vi "DSF.Shared.Configuration.Framework.New Transfer.vi"(8 "error in (no error)":errorcluster, 11 "Framework Configuration in":refnum<class "DSF.Shared.Configuration.Framework.lvclass">) -> (0 "error out":errorcluster, 2 "Transfer Configuration":refnum<class "DSF.Shared.Configuration.Transfer.lvclass">, 3 "Framework Configuration out":refnum<class "DSF.Shared.Configuration.Framework.lvclass">)   [LabVIEW 2016, in "DSF.Shared.lvlib" / "DSF.Shared.Configuration.Framework.lvclass"]
uses:
  DSF.Shared.Configuration.Framework.lvclass
  Transfer/DSF.Shared.Configuration.Transfer.lvclass
  DSF.Shared.Configuration.Framework.lvclass/DSF.Shared.Configuration.Framework.ctl
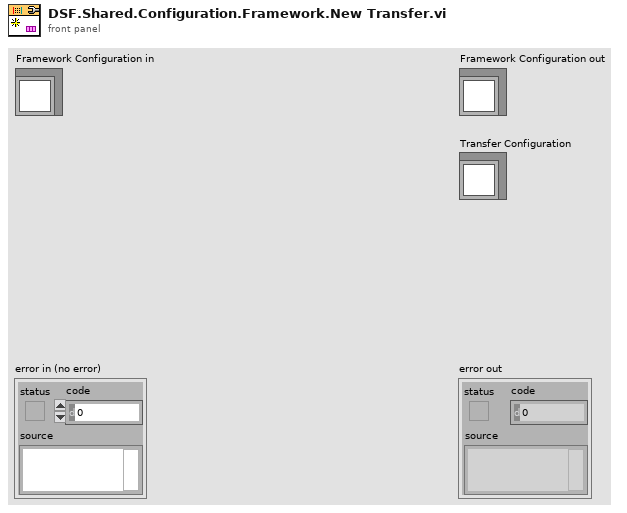
[diagram p1: front panel]
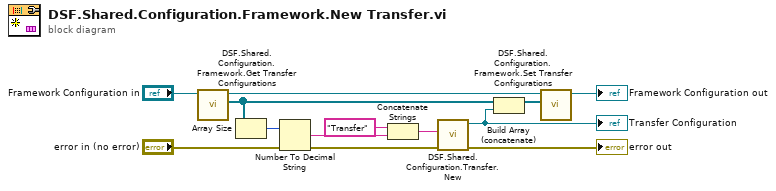
[diagram p0: block diagram]
diagram:
  n1 = call "DSF.Shared.Configuration.Framework.Get Transfer Configurations.vi"("Framework Configuration in"="Framework Configuration in") -> ("Transfer Configurations"=w4:refnum<class "DSF.Shared.Configuration.Transfer.lvclass">[], "Framework Configuration out"=w10:refnum<class "DSF.Shared.Configuration.Framework.lvclass">)  [unwired: 9 in]
  n2 = Array Size(array=w4) -> (size(s)=w3:i32)
  n3 = Number To Decimal String(number=w3) -> (decimal integer string=w2:string)  [unwired: 1 in]
  n4 = Concatenate Strings("Transfer" ("name"), w2) -> (w1:string)
  n5 = call "DSF.Shared.Configuration.Transfer.New.vi"("error in (no error)"="error in (no error)", "name"=w1) -> ("error out"=→"error out":errorcluster, "Transfer Configuration out"=w6:refnum<class "DSF.Shared.Configuration.Transfer.lvclass">)  [unwired: 8 in]
  "Transfer Configuration" <- w6
  n6 = Build Array (concatenate)(w4, w6) -> (w7:refnum<class "DSF.Shared.Configuration.Transfer.lvclass">[])
  n7 = call "DSF.Shared.Configuration.Framework.Set Transfer Configurations.vi"("Transfer Configurations"=w7, "Framework Configuration in"=w10) -> ("Framework Configuration out"=→"Framework Configuration out":refnum<class "DSF.Shared.Configuration.Framework.lvclass">)  [unwired: 9 in]
